vi "Auton Commands.vi"(7 "Roll":dbl, 8 "Turn Angle":dbl, 9 "Distance":dbl=120.0, 10 "Task":u16(ring) items=["Forward", "Backward", "Turn", "Shoot", "Turn Angle", "Roll G", "Roll L"]) -> ()   [LabVIEW 2015]
uses:
  <vilib>/Rock Robotics/Network Tables/NT Read Number.vi
  <vilib>/Rock Robotics/WPI/Utilities/WPI_GetSetVariantRefNum.vi
  <vilib>/addons/control/pid/pid.llb/PID (DBL).vi
  <vilib>/Rock Robotics/Network Tables/NT Write Number.vi
  Robot Global Data.vi
  <vilib>/addons/control/pid/NI_PID_pid.lvlib
  navX Library v2/navX Library v2.lvlib
panel:
  out "Yaw":dbl(graph)
  out "E1 Rate":dbl
  out "E2 Rate":dbl
  in  "Yaw Gains":T1={"proportional gain (Kc)"=0.2, "integral time (Ti, min)"=0.0, "derivative time (Td, min)"=0.0} {"derivative time (Td, min)" format="%.3f"; "integral time (Ti, min)" format="%.3f"; "proportional gain (Kc)" format="%.3f"}
  in  "Speed Gains":T1={"proportional gain (Kc)"=0.65, "integral time (Ti, min)"=0.001, "derivative time (Td, min)"=0.001} {"derivative time (Td, min)" format="%.3f"; "integral time (Ti, min)" format="%.3f"; "proportional gain (Kc)" format="%.3f"}
  in  "Single Turn Gains":T1={"proportional gain (Kc)"=0.12, "integral time (Ti, min)"=0.0, "derivative time (Td, min)"=0.0} {"derivative time (Td, min)" format="%.3f"; "integral time (Ti, min)" format="%.3f"; "proportional gain (Kc)" format="%.3f"}
  out "Right Motor Speed":dbl(graph)
  out "Left Motor Speed":dbl(graph)
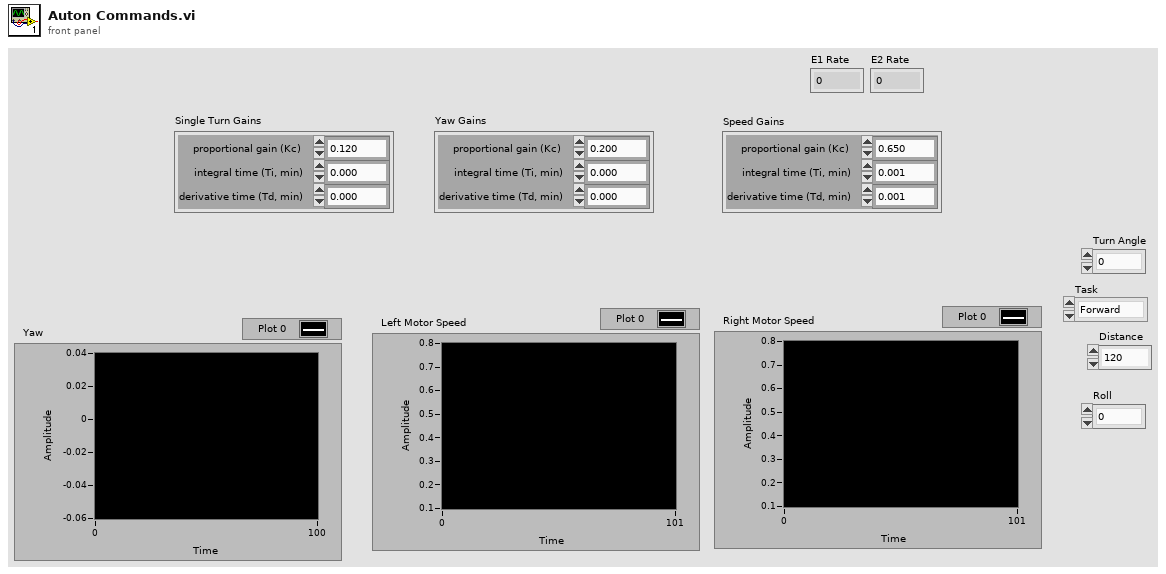
[diagram p1: front panel]
types:
  T1 = cluster{"proportional gain (Kc)":dbl, "integral time (Ti, min)":dbl, "derivative time (Td, min)":dbl}
  T2 = typedef "navX Library v2.lvlib/Z900_navX_DeviceTypeDef.ctl" = cluster{"Interface":cluster{"Protocol":T3, "Update Rate (4Hz-60Hz)":u8, "navX Open TypeDef":variant}, "Notify Packet":refnum<notifier>, "Loop VI Refnum":refnum<vi>, "Ready to Close Occurrence Refnum":refnum<k4>}
  T3 = typedef "navX Library v2.lvlib/Z900_navX_ProtocolTypeDef.ctl" = enum16{"SERIAL", "I2C", "SPI"}
  T4 = typedef "WPI_EncoderDevRef.ctl" = cluster{"DevStatus":errorcluster, "EncoderIndex":T5, "CounterIndex":T6, "DistancePerCount":dbl, "Decoding Type":T7}
  T5 = typedef "FPGA_EncoderIdx.ctl" = enum8{"Enc 0", "Enc 1", "Enc 2", "Enc 3", "Enc 4", "Enc 5", "Enc 6", "Enc 7", "Invalid"}
  T6 = typedef "FPGA_CounterCtrSystemIndex.ctl" = enum8{"Ctr 0", "Ctr 1", "Ctr 2", "Ctr 3", "Ctr 4", "Ctr 5", "Ctr 6", "Ctr 7", "Invalid"}
  T7 = typedef "WPI_EncoderType.ctl" = enum16{"1x", "2x", "4x"}
  T8 = cluster{"Yaw":dbl, "Roll":dbl, "Pitch":dbl, "Heading":dbl, "Fused Heading":dbl}
  T9 = typedef "WPI_RobotDriveDevRef.ctl" = cluster{"DevStatus":errorcluster, "Motors[]":T10[], "Square Inputs":bool, "Max Output":dbl}
  T10 = typedef "WPI_MotorControlDeviceRef.ctl" = cluster{"DeviceStatus":errorcluster, "Type":T11, "PWM":cluster{"PWM Channel":T12, "DeadBand":T13}, "CAN":cluster{"Device Number":u8, "Control Mode":T14, "Semaphore":T15, "Max Vout":dbl, "TalonSRX Control Mode":T16}, "Invert":bool}
  T11 = typedef "WPI_MotorControlType.ctl" = enum16{"PWM", "CAN", "CANTalonSRX"}
  T12 = typedef "FPGA_DIOPWMChannel.ctl" = enum8{"PWM 0", "PWM 1", "PWM 2", "PWM 3", "PWM 4", "PWM 5", "PWM 6", "PWM 7", "PWM 8", "PWM 9", "PWM MXP 0", "PWM MXP 1", "PWM MXP 2", "PWM MXP 3", "PWM MXP 4", "PWM MXP 5", "PWM MXP 6", "PWM MXP 7", "PWM MXP 8", "PWM MXP 9", "Invalid"}
  T13 = typedef "WPI_PWMDeadband.ctl" = cluster{"Name":string, "maxPositivePwm":i32, "minPositivePwm":i32, "centerPwm":i32, "maxNegativePwm":i32, "minNegativePwm":i32, "angularRange":u16}
  T14 = typedef "WPI_CANJaguar_ControlMode.ctl" = enum8{"Percent VBus", "Current", "Speed", "Position", "Voltage"}
  T15 = typedef "Semaphore RefNum" = refnum<k1>
  T16 = typedef "WPI_CANTalonSRX_APIControlMode.ctl" = enum8{"Percent VBus", "Speed", "Position", "Slave", "Unchanged / Invalid", "Voltage Compensation", "Current", "Motion Profile"}
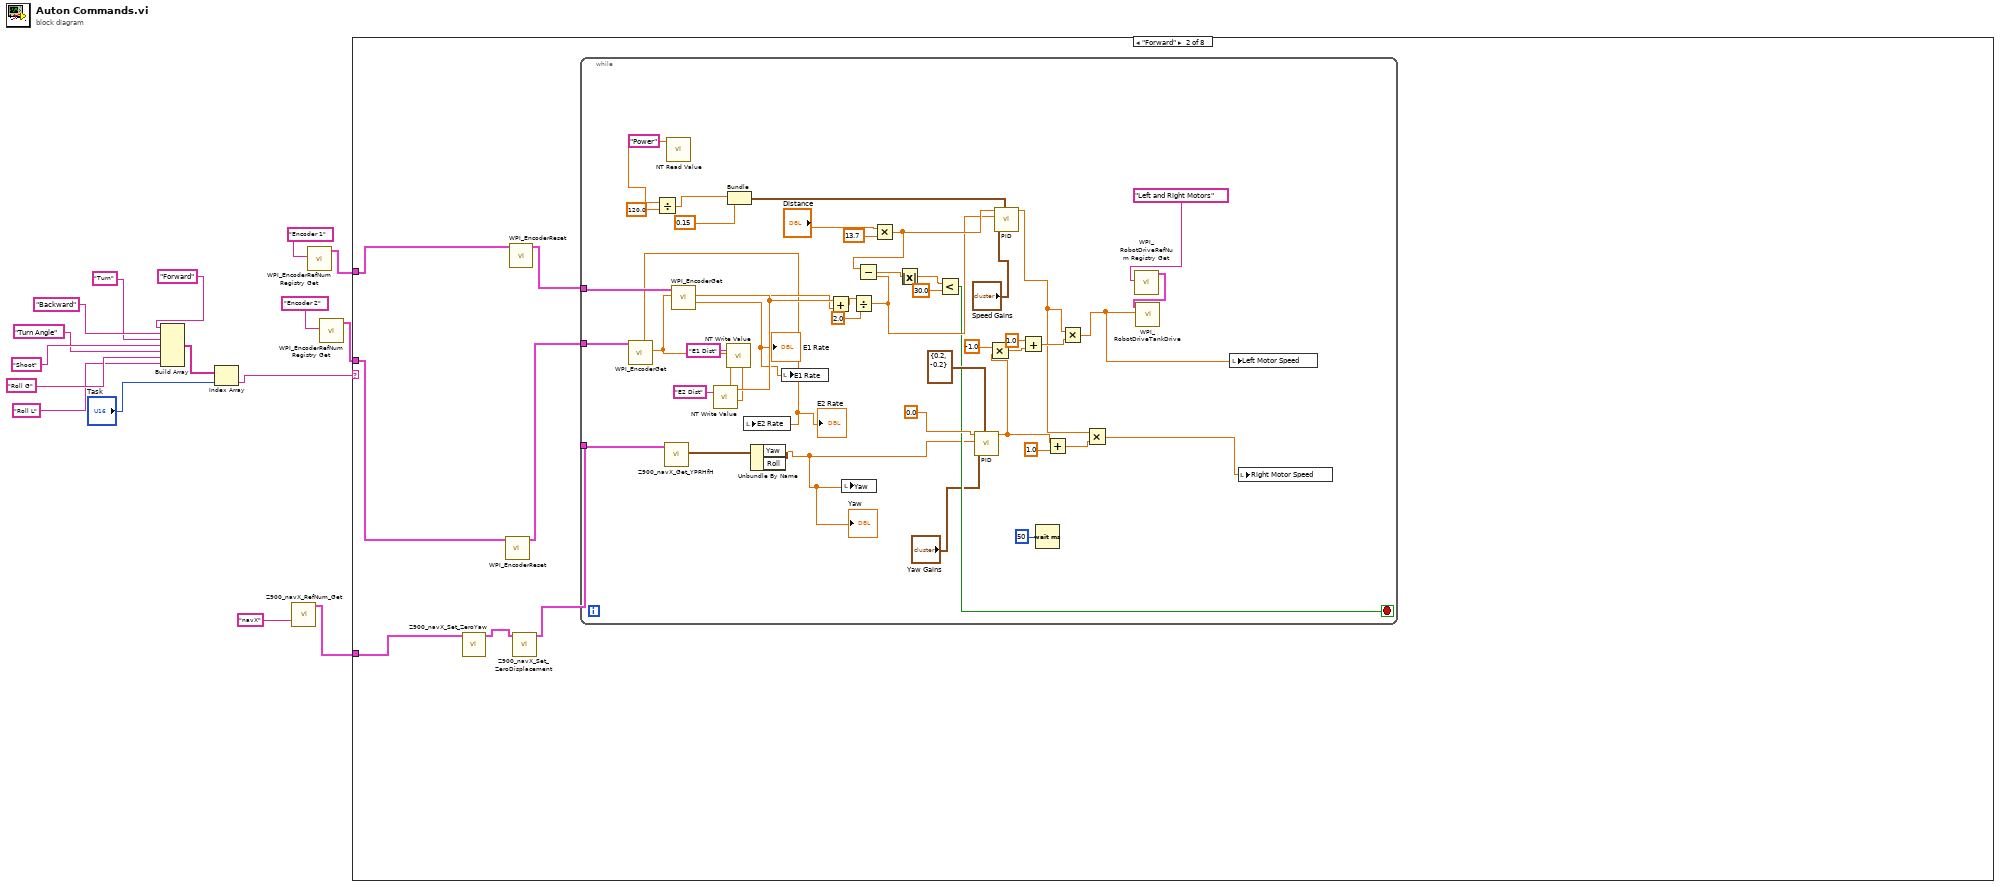
[diagram p0: block diagram]
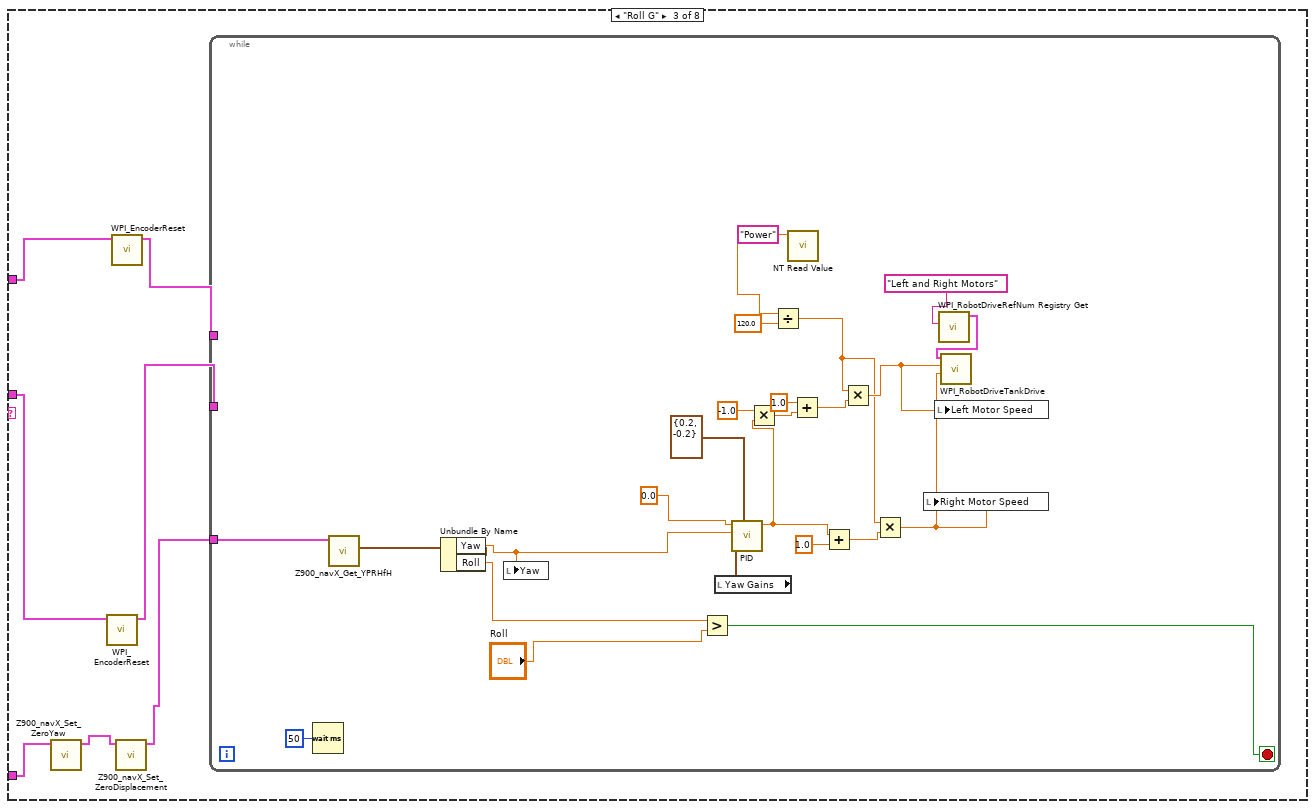
[diagram p3: hidden frame]
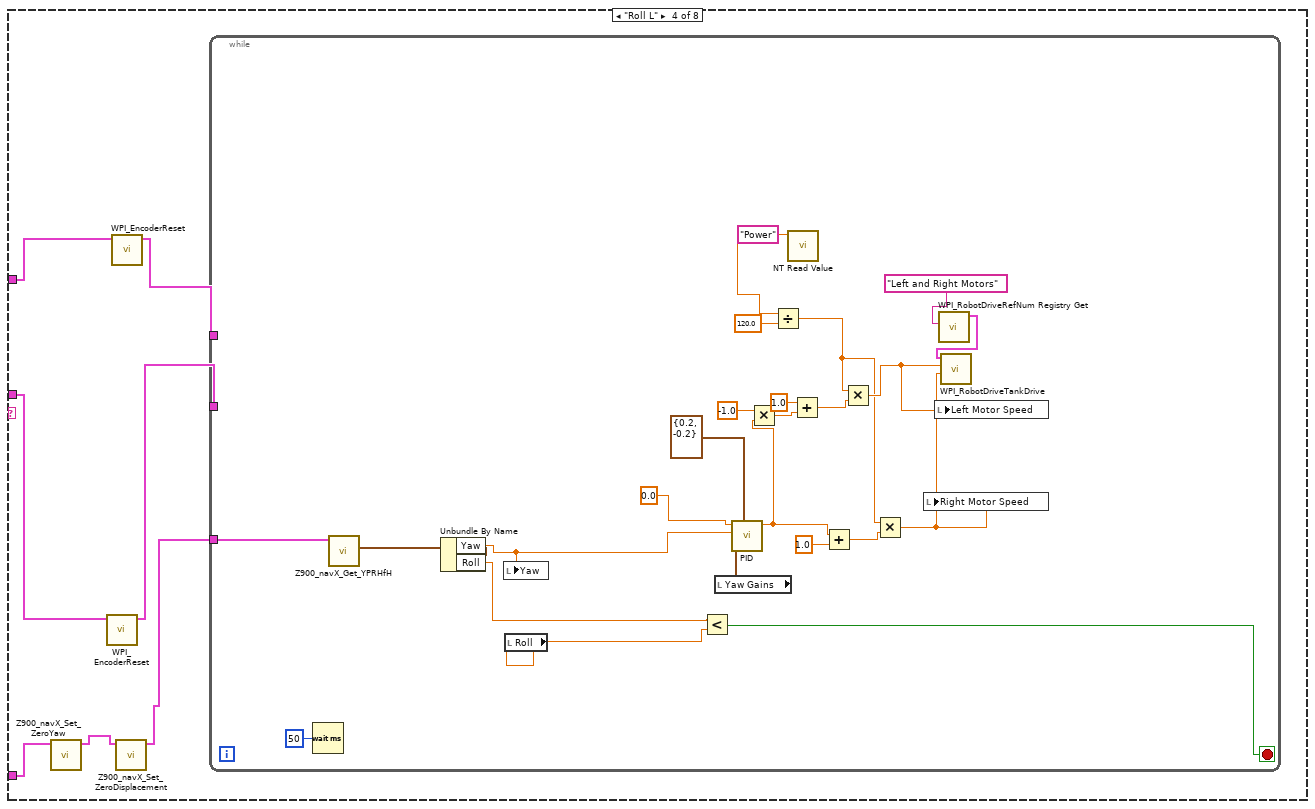
[diagram p4: hidden frame]
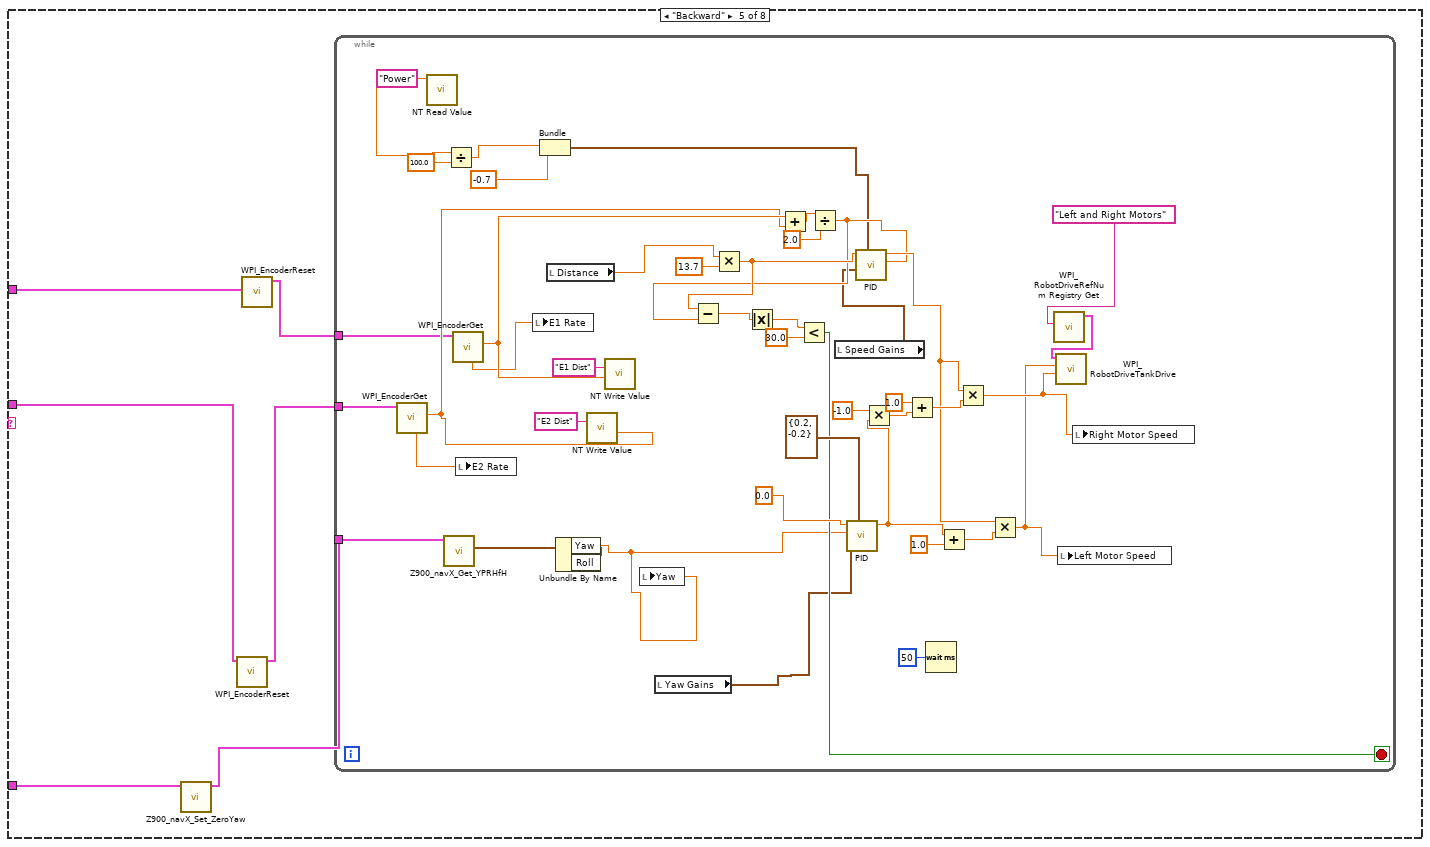
[diagram p5: hidden frame]
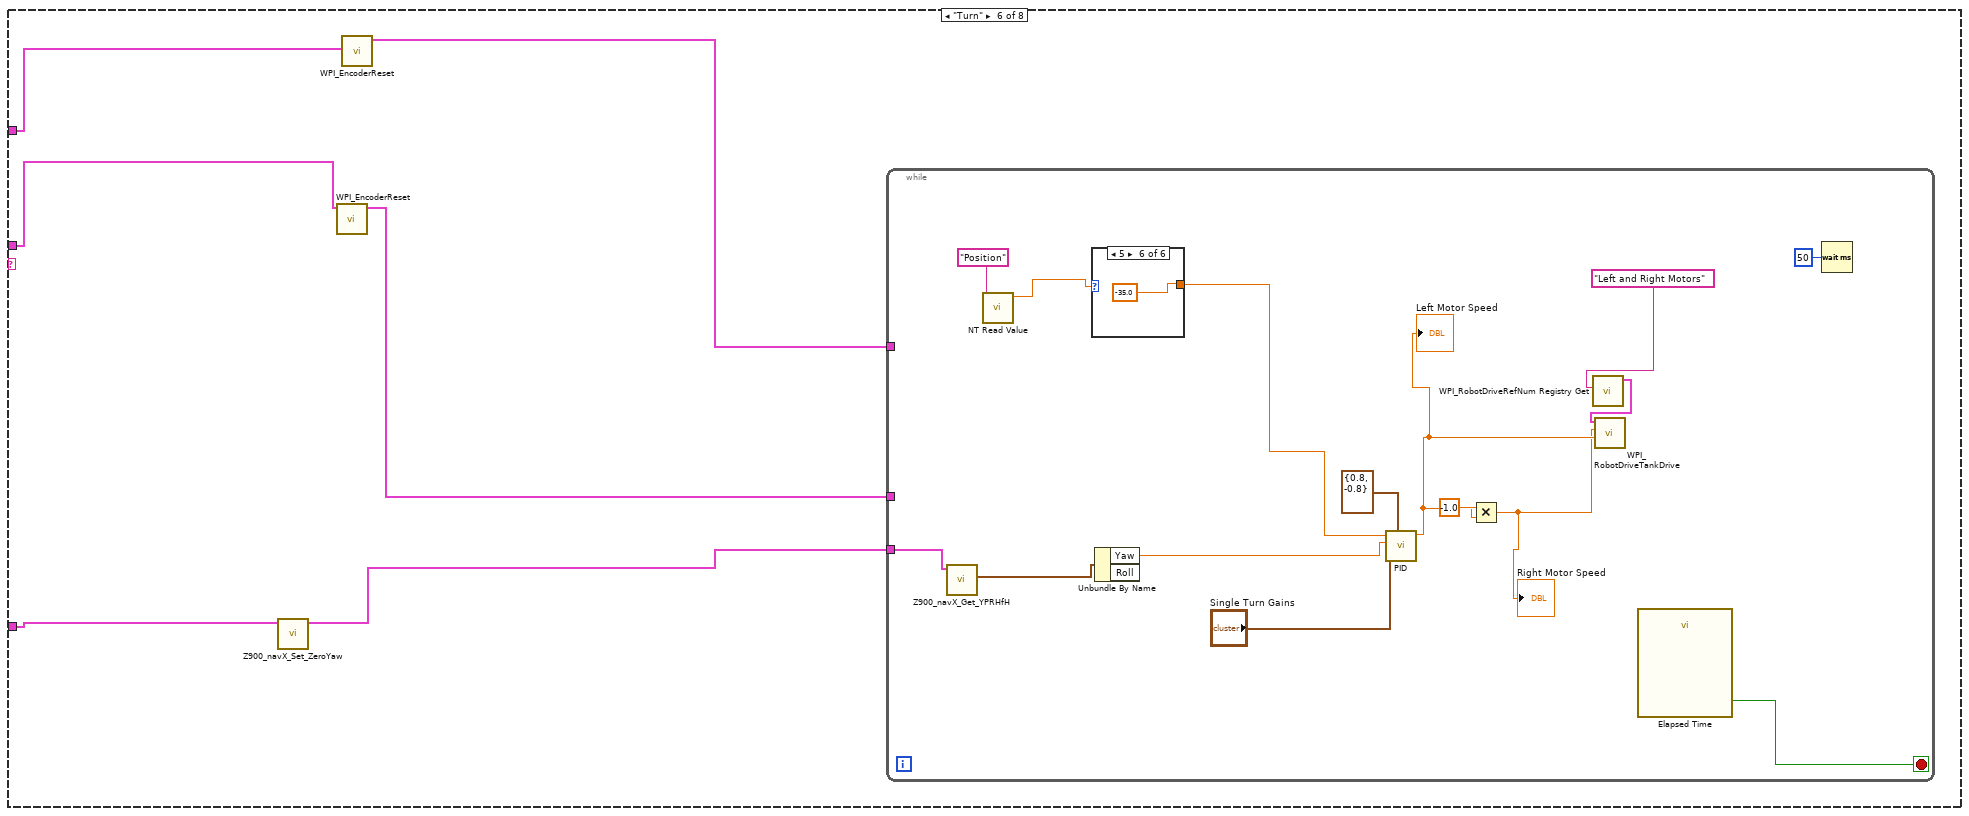
[diagram p6: hidden frame]
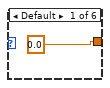
[diagram p7: hidden frame]
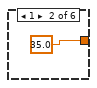
[diagram p8: hidden frame]
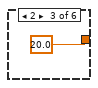
[diagram p9: hidden frame]
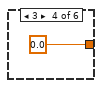
[diagram p10: hidden frame]
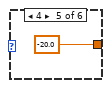
[diagram p11: hidden frame]
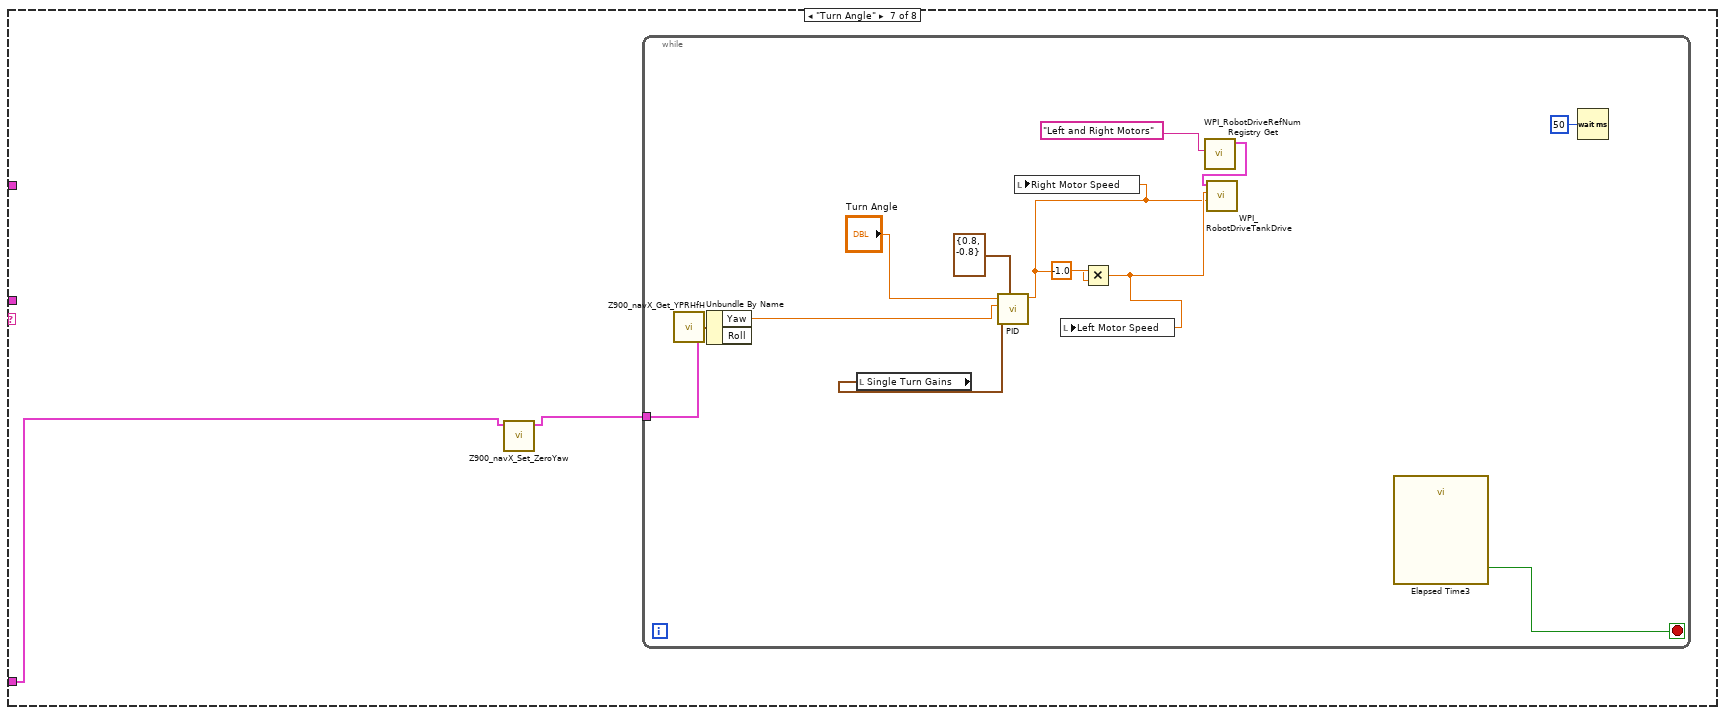
[diagram p12: hidden frame]
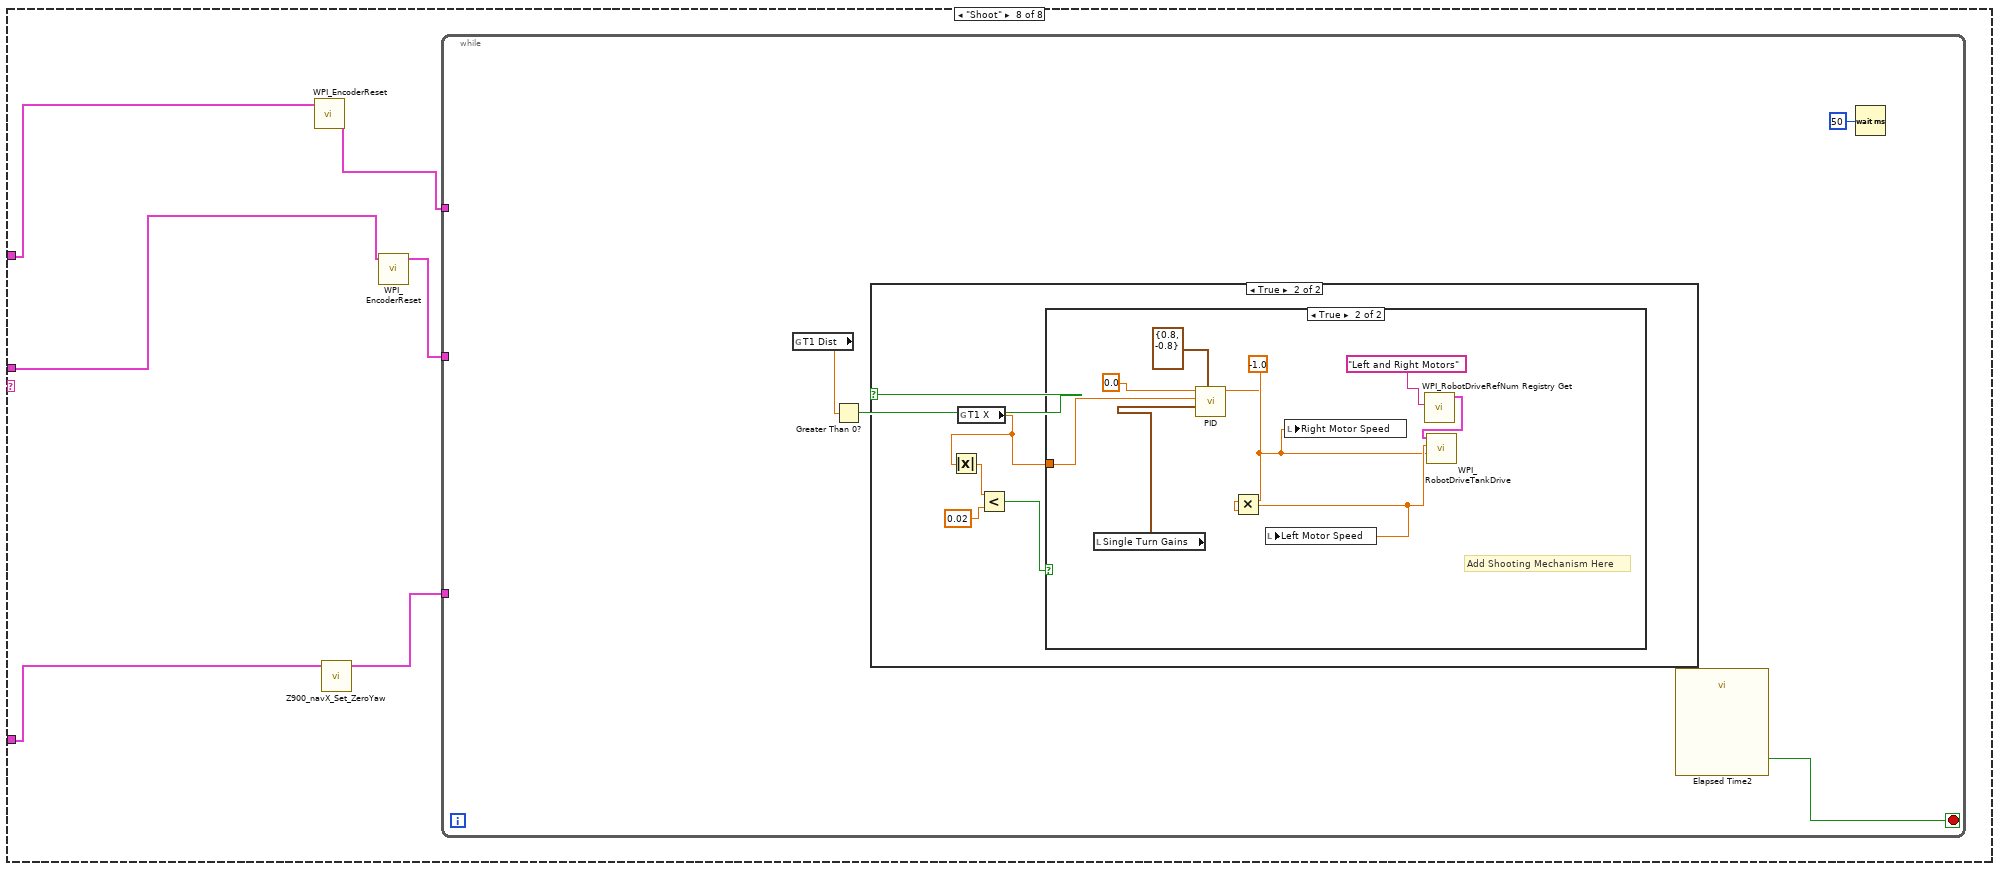
[diagram p13: hidden frame]
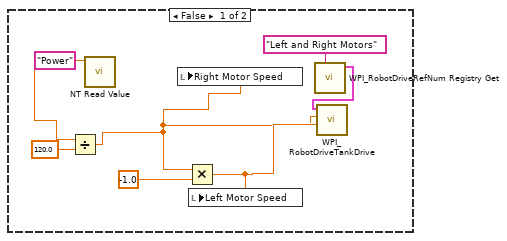
[diagram p14: hidden frame]
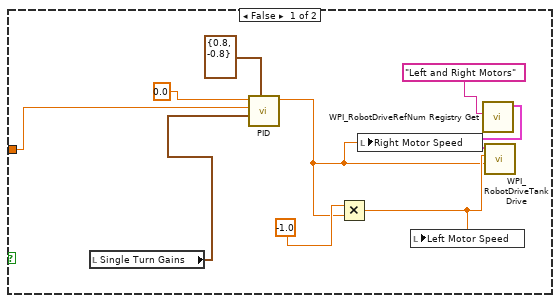
[diagram p15: hidden frame]
diagram:
  n1 = Build Array("Forward", "Backward", "Turn", "Shoot", "Turn Angle" ("element"), "Roll G" ("element"), "Roll L" ("element")) -> (w10:string[])
  n2 = Index Array(array=w10, index="Task") -> (element=w8:string)
  n3 = call "Z900_navX_RefNum_Get.vi"("refnum name"="navX") -> ("navX Device"=w11:T2)  [unwired: 9 in, 1 out]
  n4 = call <vilib>:"WPI_EncoderRefNum Registry Get.vi"("refnum name"="Encoder 1") -> ("EncoderDevRef"=w15:T4)  [unwired: 9 in, 1 out]
  n5 = call <vilib>:"WPI_EncoderRefNum Registry Get.vi"("refnum name"="Encoder 2") -> ("EncoderDevRef"=w13:T4)  [unwired: 9 in, 1 out]
  n6 = case shown="\"Forward\"" w8 {
    tunnel: w15 -> [_ w21 w73 w105 w134 w184 _ w227]
    tunnel: w13 -> [_ w20 w70 w102 w133 w183 _ w226]
    tunnel: w11 -> [_ w19 w68 w100 w132 w182 w209 w225]
    frame Default {
    }
    frame "Forward" {
      n7 = call "Z900_navX_Set_ZeroYaw.vi"("navX Device"=w19) -> ("navX Device"=w18:T2)  [unwired: 9 in, 1 out]
      n8 = call <vilib>:"WPI_EncoderReset.vi"("EncoderDevRef"=w20) -> ("EncoderDevRef"=w22:T4)  [unwired: 9 in, 1 out]
      n9 = call <vilib>:"WPI_EncoderReset.vi"("EncoderDevRef"=w21) -> ("EncoderDevRef"=w23:T4)  [unwired: 9 in, 1 out]
      n10 = call "Z900_navX_Set_ZeroDisplacement.vi"("navX Device"=w18) -> ("navX Device"=w17:T2)  [unwired: 9 in, 1 out]
      n11 = while {
        tunnel: w23 -> [w34]
        tunnel: w22 -> [w33]
        tunnel: w17 -> [w24]
        stop <- w40 stop-if-true
        n12 = call <vilib>:"WPI_EncoderGet.vi"("EncoderDevRef"=w33) -> ("Distance"=w46:dbl, "Rate"=w32:dbl)  [unwired: 5 in, 4 out]
        "E2 Rate" <- w32
        n13 = call "Z900_navX_Get_YPRHfH.vi"("navX Device"=w24) -> ("YRPHfH"=w62:T8)  [unwired: 7 in, 3 out]
        n14 = call-poly <vilib>:"NT Read Value.vi"("Name"="Power") -> ("Numeric"=w39:dbl)  [unwired: 9 in, 1 out]
        n15 = Divide(x=w39, y=120.0) -> (x/y=w37:dbl)
        n16 = call <vilib>:"WPI_EncoderGet.vi"("EncoderDevRef"=w34) -> ("Distance"=w47:dbl, "Rate"=w31:dbl)  [unwired: 5 in, 4 out]
        "E1 Rate" <- w31
        n17 = call-poly <vilib>:"NT Write Value.vi"("Numeric"=w46, "Name"="E2 Dist") -> ()  [unwired: 9 in, 1 out]
        n18 = call-poly <vilib>:"NT Write Value.vi"("Numeric"=w47, "Name"="E1 Dist") -> ()  [unwired: 9 in, 1 out]
        n19 = Bundle(w37, "output low"=0.15) -> (w35:cluster{dbl, "output low":dbl})  [unwired: 1 in]
        n20 = local write "E2 Rate"(w32) -> ()
        n21 = Unbundle By Name(w62) -> ("Yaw"=w28:dbl)  [unwired: 1 out]
        "Yaw" <- w28
        n22 = local write "E1 Rate"(w31) -> ()
        n23 = Add(x=w47, y=w46) -> (x+y=w61:dbl)
        n24 = local write "Yaw"(w28) -> ()
        n25 = Divide(x=w61, y=2.0) -> (x/y=w44:dbl)
        n26 = Multiply(x="Distance", y=13.7) -> (x*y=w45:dbl)
        n27 = Subtract(x=w45, y=w44) -> (x-y=w43:dbl)
        n28 = Absolute Value(x=w43) -> (abs(x)=w42:dbl)
        n29 = Less?(x=w42, y=30.0) -> (x < y?=w40:bool)
        n30 = call-poly <vilib>:"PID.vi"("output range"=cluster{"output high":dbl, "output low":dbl} {"output high"=0.2, "output low"=-0.2}, "PID gains"="Yaw Gains", "process variable"=w28, "setpoint"=0.0) -> ("output"=w54:dbl)  [unwired: 6 in, 1 out]
        n31 = Multiply(x=-1.0, y=w54) -> (x*y=w55:dbl)
        n32 = call-poly <vilib>:"PID.vi"("output range"=w35, "PID gains"="Speed Gains", "process variable"=w44, "setpoint"=w45) -> ("output"=w51:dbl)  [unwired: 6 in, 1 out]
        n33 = Add(x=1.0, y=w55) -> (x+y=w56:dbl)
        n34 = Wait (ms)(milliseconds to wait=u32 50) -> ()  [unwired: 1 out]
        n35 = Add(x=w54, y=1.0) -> (x+y=w57:dbl)
        n36 = Multiply(x=w51, y=w56) -> (x*y=w49:dbl)
        n37 = Multiply(x=w51, y=w57) -> (x*y=w25:dbl)
        n38 = call <vilib>:"WPI_RobotDriveRefNum Registry Get.vi"("refnum name"="Left and Right Motors") -> ("RobotDriveDevRef"=w64:T9)  [unwired: 9 in, 1 out]
        n39 = call <vilib>:"WPI_RobotDriveTankDrive.vi"("Left axis value"=w49, "RobotDriveDevRef"=w64) -> ()  [unwired: 7 in, 3 out]
        n40 = local write "Left Motor Speed"(w49) -> ()
        n41 = local write "Right Motor Speed"(w25) -> ()
      }
    }
    frame "Roll G" {
      n42 = call "Z900_navX_Set_ZeroYaw.vi"("navX Device"=w68) -> ("navX Device"=w74:T2)  [unwired: 9 in, 1 out]
      n43 = call <vilib>:"WPI_EncoderReset.vi"("EncoderDevRef"=w70) -> ("EncoderDevRef"=w71:T4)  [unwired: 9 in, 1 out]
      n44 = call <vilib>:"WPI_EncoderReset.vi"("EncoderDevRef"=w73) -> ("EncoderDevRef"=w72:T4)  [unwired: 9 in, 1 out]
      n45 = call "Z900_navX_Set_ZeroDisplacement.vi"("navX Device"=w74) -> ("navX Device"=w69:T2)  [unwired: 9 in, 1 out]
      n46 = while {
        tunnel: w72 -> [_]
        tunnel: w71 -> [_]
        tunnel: w69 -> [w82]
        stop <- w76 stop-if-true
        n47 = Wait (ms)(milliseconds to wait=u32 50) -> ()  [unwired: 1 out]
        n48 = call "Z900_navX_Get_YPRHfH.vi"("navX Device"=w82) -> ("YRPHfH"=w96:T8)  [unwired: 7 in, 3 out]
        n49 = Unbundle By Name(w96) -> ("Yaw"=w80:dbl, "Roll"=w77:dbl)
        n50 = local write "Yaw"(w80) -> ()
        n51 = Greater?(x=w77, y="Roll") -> (0:w76:bool)
        n52 = local read "Yaw Gains"() -> (w81:T1)
        n53 = call-poly <vilib>:"PID.vi"("output range"=cluster{"output high":dbl, "output low":dbl} {"output high"=0.2, "output low"=-0.2}, "PID gains"=w81, "process variable"=w80, "setpoint"=0.0) -> ("output"=w90:dbl)  [unwired: 6 in, 1 out]
        n54 = Multiply(x=-1.0, y=w90) -> (x*y=w91:dbl)
        n55 = call-poly <vilib>:"NT Read Value.vi"("Name"="Power") -> ("Numeric"=w85:dbl)  [unwired: 9 in, 1 out]
        n56 = Divide(x=w85, y=120.0) -> (x/y=w79:dbl)
        n57 = Add(x=1.0, y=w91) -> (x+y=w92:dbl)
        n58 = Add(x=w90, y=1.0) -> (x+y=w93:dbl)
        n59 = Multiply(x=w79, y=w92) -> (x*y=w87:dbl)
        n60 = Multiply(x=w79, y=w93) -> (x*y=w78:dbl)
        n61 = local write "Right Motor Speed"(w78) -> ()
        n62 = local write "Left Motor Speed"(w87) -> ()
        n63 = call <vilib>:"WPI_RobotDriveRefNum Registry Get.vi"("refnum name"="Left and Right Motors") -> ("RobotDriveDevRef"=w98:T9)  [unwired: 9 in, 1 out]
        n64 = call <vilib>:"WPI_RobotDriveTankDrive.vi"("Right axis value"=w78, "Left axis value"=w87, "RobotDriveDevRef"=w98) -> ()  [unwired: 6 in, 3 out]
      }
    }
    frame "Roll L" {
      n65 = call "Z900_navX_Set_ZeroYaw.vi"("navX Device"=w100) -> ("navX Device"=w106:T2)  [unwired: 9 in, 1 out]
      n66 = call <vilib>:"WPI_EncoderReset.vi"("EncoderDevRef"=w102) -> ("EncoderDevRef"=w103:T4)  [unwired: 9 in, 1 out]
      n67 = call <vilib>:"WPI_EncoderReset.vi"("EncoderDevRef"=w105) -> ("EncoderDevRef"=w104:T4)  [unwired: 9 in, 1 out]
      n68 = call "Z900_navX_Set_ZeroDisplacement.vi"("navX Device"=w106) -> ("navX Device"=w101:T2)  [unwired: 9 in, 1 out]
      n69 = while {
        tunnel: w104 -> [_]
        tunnel: w103 -> [_]
        tunnel: w101 -> [w114]
        stop <- w108 stop-if-true
        n70 = Wait (ms)(milliseconds to wait=u32 50) -> ()  [unwired: 1 out]
        n71 = call "Z900_navX_Get_YPRHfH.vi"("navX Device"=w114) -> ("YRPHfH"=w128:T8)  [unwired: 7 in, 3 out]
        n72 = Unbundle By Name(w128) -> ("Yaw"=w112:dbl, "Roll"=w109:dbl)
        n73 = local write "Yaw"(w112) -> ()
        n74 = local read "Roll"() -> (w107:dbl)
        n75 = Less?(x=w109, y=w107) -> (x < y?=w108:bool)
        n76 = local read "Yaw Gains"() -> (w113:T1)
        n77 = call-poly <vilib>:"PID.vi"("output range"=cluster{"output high":dbl, "output low":dbl} {"output high"=0.2, "output low"=-0.2}, "PID gains"=w113, "process variable"=w112, "setpoint"=0.0) -> ("output"=w122:dbl)  [unwired: 6 in, 1 out]
        n78 = Multiply(x=-1.0, y=w122) -> (x*y=w123:dbl)
        n79 = call-poly <vilib>:"NT Read Value.vi"("Name"="Power") -> ("Numeric"=w117:dbl)  [unwired: 9 in, 1 out]
        n80 = Divide(x=w117, y=120.0) -> (x/y=w111:dbl)
        n81 = Add(x=1.0, y=w123) -> (x+y=w124:dbl)
        n82 = Add(x=w122, y=1.0) -> (x+y=w125:dbl)
        n83 = Multiply(x=w111, y=w124) -> (x*y=w119:dbl)
        n84 = Multiply(x=w111, y=w125) -> (x*y=w110:dbl)
        n85 = local write "Right Motor Speed"(w110) -> ()
        n86 = local write "Left Motor Speed"(w119) -> ()
        n87 = call <vilib>:"WPI_RobotDriveRefNum Registry Get.vi"("refnum name"="Left and Right Motors") -> ("RobotDriveDevRef"=w130:T9)  [unwired: 9 in, 1 out]
        n88 = call <vilib>:"WPI_RobotDriveTankDrive.vi"("Right axis value"=w110, "Left axis value"=w119, "RobotDriveDevRef"=w130) -> ()  [unwired: 6 in, 3 out]
      }
    }
    frame "Backward" {
      n89 = call "Z900_navX_Set_ZeroYaw.vi"("navX Device"=w132) -> ("navX Device"=w135:T2)  [unwired: 9 in, 1 out]
      n90 = call <vilib>:"WPI_EncoderReset.vi"("EncoderDevRef"=w133) -> ("EncoderDevRef"=w136:T4)  [unwired: 9 in, 1 out]
      n91 = call <vilib>:"WPI_EncoderReset.vi"("EncoderDevRef"=w134) -> ("EncoderDevRef"=w137:T4)  [unwired: 9 in, 1 out]
      n92 = while {
        tunnel: w137 -> [w149]
        tunnel: w136 -> [w148]
        tunnel: w135 -> [w147]
        stop <- w155 stop-if-true
        n93 = call <vilib>:"WPI_EncoderGet.vi"("EncoderDevRef"=w148) -> ("Distance"=w161:dbl, "Rate"=w143:dbl)  [unwired: 5 in, 4 out]
        n94 = call-poly <vilib>:"NT Read Value.vi"("Name"="Power") -> ("Numeric"=w154:dbl)  [unwired: 9 in, 1 out]
        n95 = call "Z900_navX_Get_YPRHfH.vi"("navX Device"=w147) -> ("YRPHfH"=w176:T8)  [unwired: 7 in, 3 out]
        n96 = Divide(x=w154, y=100.0) -> (x/y=w152:dbl)
        n97 = call <vilib>:"WPI_EncoderGet.vi"("EncoderDevRef"=w149) -> ("Distance"=w162:dbl, "Rate"=w142:dbl)  [unwired: 5 in, 4 out]
        n98 = local write "E2 Rate"(w143) -> ()
        n99 = local write "E1 Rate"(w142) -> ()
        n100 = Bundle(w152, "output low"=-0.7) -> (w150:cluster{dbl, "output low":dbl})  [unwired: 1 in]
        n101 = local read "Distance"() -> (w141:dbl)
        n102 = Unbundle By Name(w176) -> ("Yaw"=w145:dbl)  [unwired: 1 out]
        n103 = call-poly <vilib>:"NT Write Value.vi"("Numeric"=w161, "Name"="E2 Dist") -> ()  [unwired: 9 in, 1 out]
        n104 = call-poly <vilib>:"NT Write Value.vi"("Numeric"=w162, "Name"="E1 Dist") -> ()  [unwired: 9 in, 1 out]
        n105 = local write "Yaw"(w145) -> ()
        n106 = local read "Yaw Gains"() -> (w144:T1)
        n107 = Multiply(x=w141, y=13.7) -> (x*y=w160:dbl)
        n108 = Add(x=w162, y=w161) -> (x+y=w175:dbl)
        n109 = Divide(x=w175, y=2.0) -> (x/y=w159:dbl)
        n110 = Subtract(x=w160, y=w159) -> (x-y=w158:dbl)
        n111 = Absolute Value(x=w158) -> (abs(x)=w157:dbl)
        n112 = Less?(x=w157, y=30.0) -> (x < y?=w155:bool)
        n113 = local read "Speed Gains"() -> (w138:T1)
        n114 = call-poly <vilib>:"PID.vi"("output range"=cluster{"output high":dbl, "output low":dbl} {"output high"=0.2, "output low"=-0.2}, "PID gains"=w144, "process variable"=w145, "setpoint"=0.0) -> ("output"=w168:dbl)  [unwired: 6 in, 1 out]
        n115 = call-poly <vilib>:"PID.vi"("output range"=w150, "PID gains"=w138, "process variable"=w159, "setpoint"=w160) -> ("output"=w165:dbl)  [unwired: 6 in, 1 out]
        n116 = Multiply(x=-1.0, y=w168) -> (x*y=w169:dbl)
        n117 = Add(x=1.0, y=w169) -> (x+y=w170:dbl)
        n118 = Wait (ms)(milliseconds to wait=u32 50) -> ()  [unwired: 1 out]
        n119 = Add(x=w168, y=1.0) -> (x+y=w171:dbl)
        n120 = Multiply(x=w165, y=w170) -> (x*y=w140:dbl)
        n121 = Multiply(x=w165, y=w171) -> (x*y=w139:dbl)
        n122 = call <vilib>:"WPI_RobotDriveRefNum Registry Get.vi"("refnum name"="Left and Right Motors") -> ("RobotDriveDevRef"=w178:T9)  [unwired: 9 in, 1 out]
        n123 = call <vilib>:"WPI_RobotDriveTankDrive.vi"("Right axis value"=w140, "Left axis value"=w139, "RobotDriveDevRef"=w178) -> ()  [unwired: 6 in, 3 out]
        n124 = local write "Left Motor Speed"(w139) -> ()
        n125 = local write "Right Motor Speed"(w140) -> ()
      }
    }
    frame "Turn" {
      n126 = call "Z900_navX_Set_ZeroYaw.vi"("navX Device"=w182) -> ("navX Device"=w185:T2)  [unwired: 9 in, 1 out]
      n127 = call <vilib>:"WPI_EncoderReset.vi"("EncoderDevRef"=w183) -> ("EncoderDevRef"=w186:T4)  [unwired: 9 in, 1 out]
      n128 = call <vilib>:"WPI_EncoderReset.vi"("EncoderDevRef"=w184) -> ("EncoderDevRef"=w187:T4)  [unwired: 9 in, 1 out]
      n129 = while {
        tunnel: w187 -> [_]
        tunnel: w186 -> [_]
        tunnel: w185 -> [w198]
        stop <- w194 stop-if-true
        n130 = call "Z900_navX_Get_YPRHfH.vi"("navX Device"=w198) -> ("YRPHfH"=w197:T8)  [unwired: 7 in, 3 out]
        n131 = call-poly <vilib>:"NT Read Value.vi"("Name"="Position") -> ("Numeric"=w191:dbl)  [unwired: 9 in, 1 out]
        n132 = case shown="5" w191 {
          tunnel: [0.0 35.0 20.0 0.0 -20.0 -35.0] -> w192
          frame Default {
          }
          frame 1 {
          }
          frame 2 {
          }
          frame 3 {
          }
          frame 4 {
          }
          frame 5 {
          }
        }
        n133 = Unbundle By Name(w197) -> ("Yaw"=w195:dbl)  [unwired: 1 out]
        n134 = call-poly <vilib>:"PID.vi"("output range"=cluster{"output high":dbl, "output low":dbl} {"output high"=0.8, "output low"=-0.8}, "PID gains"="Single Turn Gains", "process variable"=w195, "setpoint"=w192) -> ("output"=w189:dbl)  [unwired: 6 in, 1 out]
        "Left Motor Speed" <- w189
        n135 = Multiply(x=-1.0, y=w189) -> (x*y=w188:dbl)
        "Right Motor Speed" <- w188
        n136 = call <vilib>:"WPI_RobotDriveRefNum Registry Get.vi"("refnum name"="Left and Right Motors") -> ("RobotDriveDevRef"=w201:T9)  [unwired: 9 in, 1 out]
        n137 = call <vilib>:"WPI_RobotDriveTankDrive.vi"("Right axis value"=w189, "Left axis value"=w188, "RobotDriveDevRef"=w201) -> ()  [unwired: 6 in, 3 out]
        n138 = call "Elapsed Time"() -> ("Time has Elapsed"=w194:bool)  [unwired: 12 in, 7 out]
        n139 = Wait (ms)(milliseconds to wait=u32 50) -> ()  [unwired: 1 out]
      }
    }
    frame "Turn Angle" {
      n140 = call "Z900_navX_Set_ZeroYaw.vi"("navX Device"=w209) -> ("navX Device"=w210:T2)  [unwired: 9 in, 1 out]
      n141 = while {
        tunnel: w210 -> [w219]
        stop <- w215 stop-if-true
        n142 = call "Z900_navX_Get_YPRHfH.vi"("navX Device"=w219) -> ("YRPHfH"=w218:T8)  [unwired: 7 in, 3 out]
        n143 = Unbundle By Name(w218) -> ("Yaw"=w216:dbl)  [unwired: 1 out]
        n144 = local read "Single Turn Gains"() -> (w213:T1)
        n145 = call-poly <vilib>:"PID.vi"("output range"=cluster{"output high":dbl, "output low":dbl} {"output high"=0.8, "output low"=-0.8}, "PID gains"=w213, "process variable"=w216, "setpoint"="Turn Angle") -> ("output"=w211:dbl)  [unwired: 6 in, 1 out]
        n146 = local write "Right Motor Speed"(w211) -> ()
        n147 = Multiply(x=-1.0, y=w211) -> (x*y=w212:dbl)
        n148 = local write "Left Motor Speed"(w212) -> ()
        n149 = call <vilib>:"WPI_RobotDriveRefNum Registry Get.vi"("refnum name"="Left and Right Motors") -> ("RobotDriveDevRef"=w222:T9)  [unwired: 9 in, 1 out]
        n150 = call <vilib>:"WPI_RobotDriveTankDrive.vi"("Right axis value"=w211, "Left axis value"=w212, "RobotDriveDevRef"=w222) -> ()  [unwired: 6 in, 3 out]
        n151 = call "Elapsed Time3"() -> ("Time has Elapsed"=w215:bool)  [unwired: 12 in, 7 out]
        n152 = Wait (ms)(milliseconds to wait=u32 50) -> ()  [unwired: 1 out]
      }
    }
    frame "Shoot" {
      n153 = call <vilib>:"WPI_EncoderReset.vi"("EncoderDevRef"=w227) -> ("EncoderDevRef"=w224:T4)  [unwired: 9 in, 1 out]
      n154 = call "Z900_navX_Set_ZeroYaw.vi"("navX Device"=w225) -> ("navX Device"=w228:T2)  [unwired: 9 in, 1 out]
      n155 = call <vilib>:"WPI_EncoderReset.vi"("EncoderDevRef"=w226) -> ("EncoderDevRef"=w229:T4)  [unwired: 9 in, 1 out]
      n156 = while {
        tunnel: w224 -> [_]
        tunnel: w229 -> [_]
        tunnel: w228 -> [_]
        stop <- w232 stop-if-true
        n157 = global read "Robot Global Data.vi" "T1 Dist"() -> (w231:dbl)
        n158 = Greater Than 0?(x=w231) -> (x > 0?=w230:bool)
        n159 = case shown="True" w230 {
          frame False {
            n160 = call-poly <vilib>:"NT Read Value.vi"("Name"="Power") -> ("Numeric"=w238:dbl)  [unwired: 9 in, 1 out]
            n161 = Divide(x=w238, y=120.0) -> (x/y=w234:dbl)
            n162 = local write "Right Motor Speed"(w234) -> ()
            n163 = Multiply(x=w234, y=-1.0) -> (x*y=w235:dbl)
            n164 = local write "Left Motor Speed"(w235) -> ()
            n165 = call <vilib>:"WPI_RobotDriveRefNum Registry Get.vi"("refnum name"="Left and Right Motors") -> ("RobotDriveDevRef"=w240:T9)  [unwired: 9 in, 1 out]
            n166 = call <vilib>:"WPI_RobotDriveTankDrive.vi"("Right axis value"=w235, "Left axis value"=w234, "RobotDriveDevRef"=w240) -> ()  [unwired: 6 in, 3 out]
          }
          frame True {
            n167 = global read "Robot Global Data.vi" "T1 X"() -> (w245:dbl)
            n168 = Absolute Value(x=w245) -> (abs(x)=w244:dbl)
            n169 = Less?(x=w244, y=0.02) -> (x < y?=w242:bool)
            n170 = case shown="True" w242 {
              tunnel: w245 -> [w249 w258]
              frame False {
                n171 = local read "Single Turn Gains"() -> (w248:T1)
                n172 = call-poly <vilib>:"PID.vi"("output range"=cluster{"output high":dbl, "output low":dbl} {"output high"=0.8, "output low"=-0.8}, "PID gains"=w248, "process variable"=w249, "setpoint"=0.0) -> ("output"=w246:dbl)  [unwired: 6 in, 1 out]
                n173 = Multiply(x=-1.0, y=w246) -> (x*y=w247:dbl)
                n174 = local write "Right Motor Speed"(w246) -> ()
                n175 = local write "Left Motor Speed"(w247) -> ()
                n176 = call <vilib>:"WPI_RobotDriveRefNum Registry Get.vi"("refnum name"="Left and Right Motors") -> ("RobotDriveDevRef"=w252:T9)  [unwired: 9 in, 1 out]
                n177 = call <vilib>:"WPI_RobotDriveTankDrive.vi"("Right axis value"=w246, "Left axis value"=w247, "RobotDriveDevRef"=w252) -> ()  [unwired: 6 in, 3 out]
              }
              frame True {
                # "Add Shooting Mechanism Here"
                n178 = local read "Single Turn Gains"() -> (w257:T1)
                n179 = call-poly <vilib>:"PID.vi"("output range"=cluster{"output high":dbl, "output low":dbl} {"output high"=0.8, "output low"=-0.8}, "PID gains"=w257, "process variable"=w258, "setpoint"=0.0) -> ("output"=w255:dbl)  [unwired: 6 in, 1 out]
                n180 = Multiply(x=-1.0, y=w255) -> (x*y=w256:dbl)
                n181 = local write "Left Motor Speed"(w256) -> ()
                n182 = local write "Right Motor Speed"(w255) -> ()
                n183 = call <vilib>:"WPI_RobotDriveRefNum Registry Get.vi"("refnum name"="Left and Right Motors") -> ("RobotDriveDevRef"=w261:T9)  [unwired: 9 in, 1 out]
                n184 = call <vilib>:"WPI_RobotDriveTankDrive.vi"("Right axis value"=w255, "Left axis value"=w256, "RobotDriveDevRef"=w261) -> ()  [unwired: 6 in, 3 out]
              }
            }
          }
        }
        n185 = call "Elapsed Time2"() -> ("Time has Elapsed"=w232:bool)  [unwired: 12 in, 7 out]
        n186 = Wait (ms)(milliseconds to wait=u32 50) -> ()  [unwired: 1 out]
      }
    }
  }
